vi "UpdatePressure3.vi"(6 "Transducer (psi)":dbl(ring)=1.0 items=["+/- .18 psi"=1.0, "+/- .36 psi"=2.0, "+/- 1.08 psi"=3.0], 9 "PressureOffset":dbl, 10 "Arduino error in":errorcluster, 11 "ArduinoHandle":T1={"VISA resource"="", "Board Type"=enum."Uno", "Connection Type"=enum."USB / Serial", "Bytes Per Packet (15)"=15}) -> (2 "Arduino error out":errorcluster, 3 "Pressure (psi)":dbl)   [LabVIEW 2011]
uses:
  <vilib>/LabVIEW Interface for Arduino/Type Defs/Arduino Resource.ctl
  <vilib>/LabVIEW Interface for Arduino/Type Defs/Board Type.ctl
  <vilib>/LabVIEW Interface for Arduino/LabVIEW Interface for Arduino.lvlib
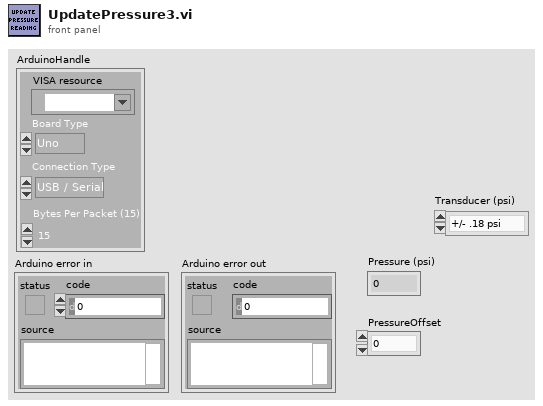
[diagram p1: front panel]
types:
  T1 = typedef "LabVIEW Interface for Arduino.lvlib/Arduino Resource.ctl" = cluster{"VISA resource":refnum<visa-resource-name>, "Board Type":T2, "Connection Type":enum8{"USB / Serial"}, "Bytes Per Packet (15)":u8}
  T2 = typedef "LabVIEW Interface for Arduino.lvlib/Board Type.ctl" = enum16{"Uno", "Dimuelanove w/Atmega 328", "Mega 2560"}
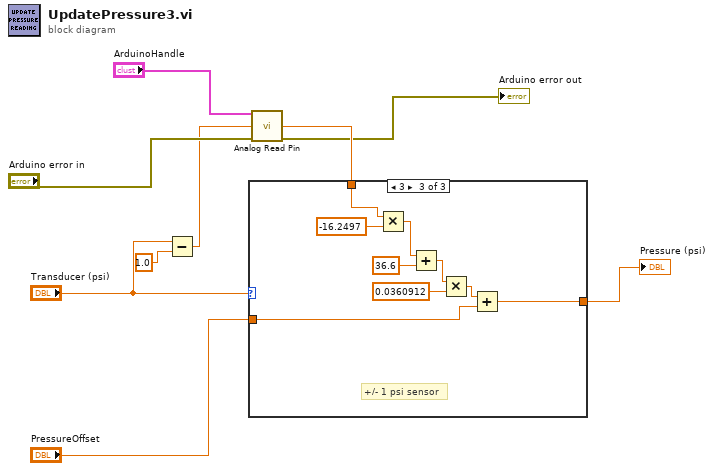
[diagram p0: block diagram]
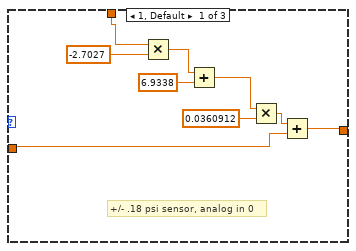
[diagram p2: hidden frame]
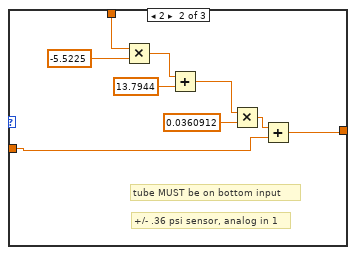
[diagram p3: hidden frame]
diagram:
  n1 = Subtract(x="Transducer (psi)", y=1.0) -> (x-y=w1:dbl)
  n2 = call <vilib>:"Analog Read Pin.vi"("Arduino Resource"="ArduinoHandle", "Analog Input Pin (0)"=w1, "error in"="Arduino error in") -> ("Voltage"=w9:dbl, "error out"=→"Arduino error out":errorcluster)  [unwired: 10 in, 1 out]
  n3 = case shown="3" "Transducer (psi)" {
    tunnel: w9 -> [w12 w23 w30]
    tunnel: "PressureOffset" -> [w10 w25 w29]
    tunnel: [w11 w24 w28] -> w4
    frame 1, Default {
      # "+/- .18 psi sensor, analog in 0"
      n4 = Multiply(x=w12, y=-2.7027) -> (x*y=w15:dbl)
      n5 = Add(x=w15, y=6.9338) -> (x+y=w13:dbl)
      n6 = Multiply(x=w13, y=0.0360912) -> (x*y=w17:dbl)
      n7 = Add(x=w17, y=w10) -> (x+y=w11:dbl)
    }
    frame 2 {
      # "tube MUST be on bottom input"
      # "+/- .36 psi sensor, analog in 1"
      n8 = Multiply(x=w23, y=-5.5225) -> (x*y=w21:dbl)
      n9 = Add(x=w21, y=13.7944) -> (x+y=w19:dbl)
      n10 = Multiply(x=w19, y=0.0360912) -> (x*y=w26:dbl)
      n11 = Add(x=w26, y=w25) -> (x+y=w24:dbl)
    }
    frame 3 {
      # "+/- 1 psi sensor"
      n12 = Multiply(x=w30, y=-16.2497) -> (x*y=w35:dbl)
      n13 = Add(x=w35, y=36.6) -> (x+y=w33:dbl)
      n14 = Multiply(x=w33, y=0.0360912) -> (x*y=w31:dbl)
      n15 = Add(x=w31, y=w29) -> (x+y=w28:dbl)
    }
  }
  "Pressure (psi)" <- w4
